vi "2039_JoystickMecanumCartesianMapping.vi"(6 "Max Output":dbl=1.0, 7 "Gyro Angle":dbl, 8 "Rotation":dbl, 9 "Y":dbl, 10 "X":dbl) -> (0 "Rear Right":dbl, 1 "Rear Left":dbl, 2 "Front Right":dbl, 3 "Front Left":dbl)   [LabVIEW 2015]
doc: "Maps the joystick inputs for holonomic driving. Holonomic driving allows you to move the robot in any direction without first rotating or maneuvering the robot.\n\nThis VI assumes the robot to have either four omni-directional wheels and four motors mounted at 45 degree angles in the four corners of a square frame or to have four mecanum wheels driven by four motors."
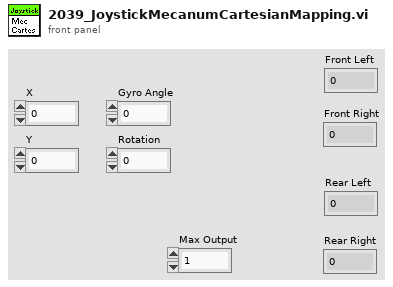
[diagram p1: front panel]
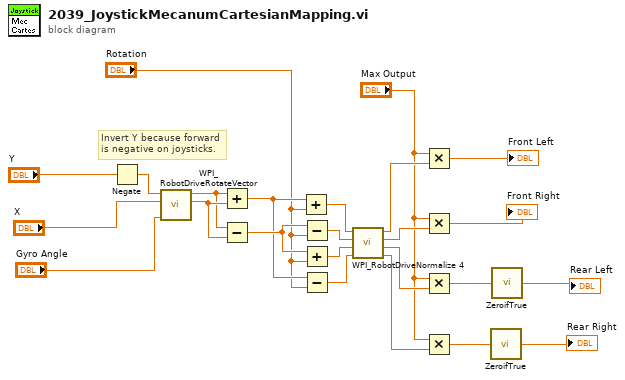
[diagram p0: block diagram]
diagram:
  # "Invert Y because forward is negative on joysticks."
  n1 = Negate(x="Y") -> (-x=w24:dbl)
  n2 = call <vilib>:"WPI_RobotDriveRotateVector.vi"("Angle"="Gyro Angle", "X"="X", "Y"=w24) -> ("X'"=w17:dbl, "Y'"=w16:dbl)  [unwired: 7 out]
  n3 = Add(x=w16, y=w17) -> (x+y=w19:dbl)
  n4 = Subtract(x=w16, y=w17) -> (x-y=w21:dbl)
  n5 = Add(x=w19, y="Rotation") -> (x+y=w23:dbl)
  n6 = Subtract(x=w21, y="Rotation") -> (x-y=w22:dbl)
  n7 = Add(x=w21, y="Rotation") -> (x+y=w20:dbl)
  n8 = Subtract(x=w19, y="Rotation") -> (x-y=w18:dbl)
  n9 = call <vilib>:"WPI_RobotDriveNormalize 4.vi"("D"=w18, "C"=w20, "B"=w22, "A"=w23) -> ("D'"=w12:dbl, "C'"=w13:dbl, "B'"=w14:dbl, "A'"=w15:dbl)
  n10 = Multiply(x="Max Output", y=w15) -> (x*y=→"Front Left":dbl)
  n11 = Multiply(x="Max Output", y=w14) -> (x*y=→"Front Right":dbl)
  n12 = Multiply(x="Max Output", y=w13) -> (x*y=w4:dbl)
  n13 = Multiply(x="Max Output", y=w12) -> (x*y=w2:dbl)
  n14 = call "ZeroifTrue.vi"("Input"=w2) -> ("Output"=→"Rear Right":dbl)
  n15 = call "ZeroifTrue.vi"("Input"=w4) -> ("Output"=→"Rear Left":dbl)
